vi "总磷总氮MB_api.vi"(6 "Slave ID":u8=1, 7 "STEP":enum16{"open", "read", "write", "close"}(ring)=enum."read", 8 "Error in":errorcluster caption="Error in (no error)", 9 "values":u16[](array[numeric]), 10 "quantity":u16, 11 "starting address":u16 format="%04xH") -> (0 "error out":errorcluster, 2 "MB session out":refnum<class "MB_Master.lvclass">, 3 "Registers":u16[](array[numeric]))   [LabVIEW 2016, in "斯坦道总磷.lvlib"]
uses:
  <vilib>/Plasmionique/MB Master/MB_Master/MB_Master.lvclass
  <vilib>/Plasmionique/MB Master/MB_Master_Serial/MB_Master_Serial.lvclass
  D:/Program Files (x86)/National Instruments/LabVIEW 2016/vi.lib/Plasmionique/MB Master/MB_Master/MB_Master.lvclass
  <vilib>/Plasmionique/MB Master/MB_Master_TCP/MB_Master_TCP.lvclass
  <vilib>/Plasmionique/MB Master/MB Master.lvlib
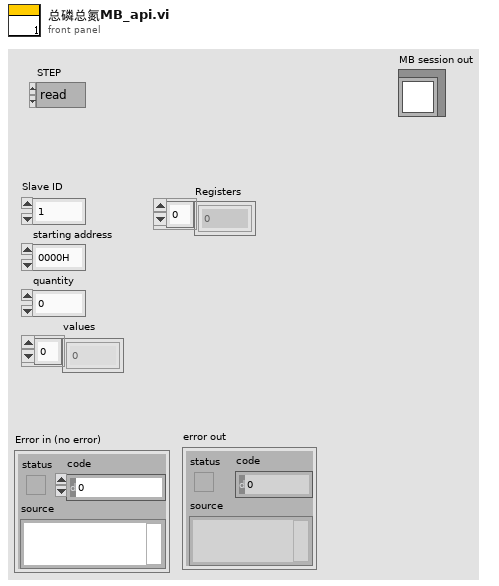
[diagram p1: front panel]
types:
  T1 = cluster{"baud rate (bps)":u32, "stop bits":u16, "parity":u16, "flow control":u16, "timeout":u32, "retries":i32}
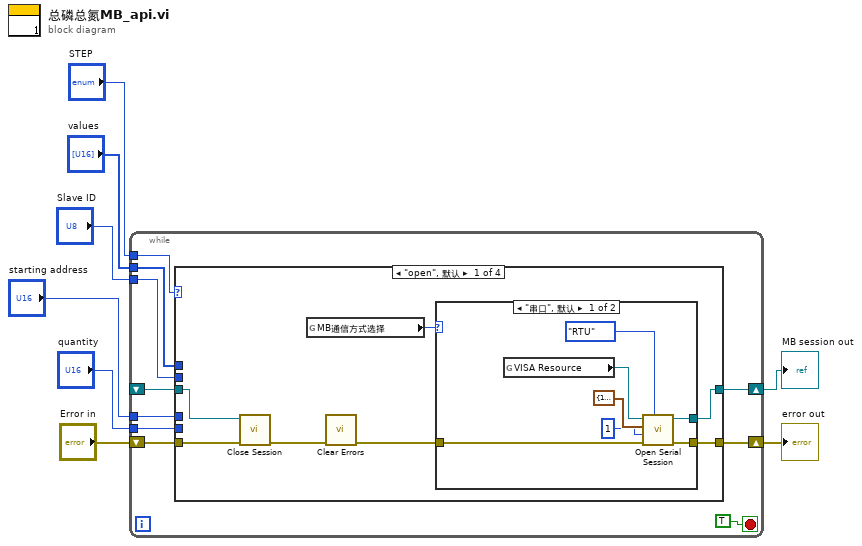
[diagram p0: block diagram]
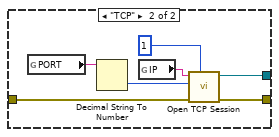
[diagram p2: hidden frame]
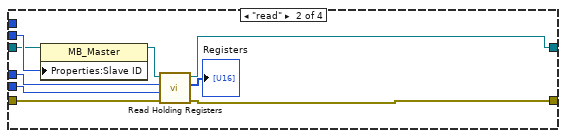
[diagram p3: hidden frame]
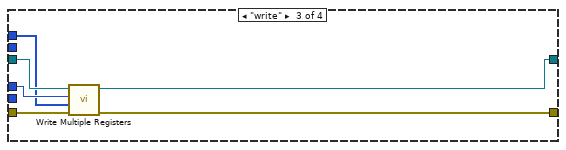
[diagram p4: hidden frame]
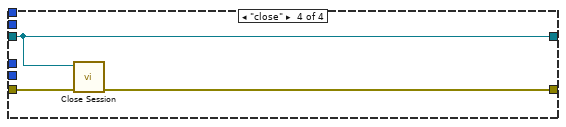
[diagram p5: hidden frame]
diagram:
  n1 = while {
    shift-right: [w9] -> w1
    shift-left: _ -> [w18]
    shift-right: [w10] -> w7
    shift-left: "Error in" -> [w17]
    tunnel: "Slave ID" -> [w16]
    tunnel: "starting address" -> [w15]
    tunnel: "quantity" -> [w14]
    tunnel: "STEP" -> [w13]
    tunnel: "values" -> [w12]
    stop <- TRUE stop-if-true
    n2 = case shown="\"open\", 默认" w13 {
      tunnel: w18 -> [w23 w41 w52 w55]
      tunnel: w17 -> [w22 w48 w54 w57]
      tunnel: [w24 w47 w51 w55] -> w9
      tunnel: [w25 w46 w53 w56] -> w10
      tunnel: w16 -> [_ w44 _ _]
      tunnel: w15 -> [_ w43 w50 _]
      tunnel: w14 -> [_ w42 _ _]
      tunnel: w12 -> [_ _ w49 _]
      frame "open", Default {
        n3 = call-dynamic "Close Session.vi"("error in (no error)"=w22, "MB session in"=w23) -> ("error out"=w21:errorcluster)  [unwired: 9 in]
        n4 = global read "总磷断电保存全局变量.vi" "MB通信方式选择"() -> (w19:enum16{"串口", "TCP"})
        n5 = call <vilib>:"Clear Errors.vi"("error in (no error)"=w21) -> ("error out"=w20:errorcluster)  [unwired: 5 in, 1 out]
        n6 = case shown="\"串口\", 默认" w19 {
          tunnel: [w30 w37] -> w25
          tunnel: [w27 w36] -> w24
          tunnel: w20 -> [w28 w38]
          frame "串口", Default {
            n7 = global read "总磷断电保存全局变量.vi" "VISA Resource"() -> (w26:refnum<visa-resource-name>)
            n8 = call <vilib>:"Open Serial Session.vi"("Mode (RTU)"=enum16{"RTU", "ASCII"}."RTU", "Error in"=w28, "Slave ID"=u8 1, "Serial Config"=T1 {"baud rate (bps)"=115200, "stop bits"=10, "parity"=0, "flow control"=0, "timeout"=1000, "retries"=1}, "VISA Resource"=w26) -> ("Error out"=w30:errorcluster, "MB_Serial session"=w27:refnum<class "MB_Master_Serial.lvclass">)  [unwired: 5 in]
          }
          frame "TCP" {
            n9 = global read "总磷断电保存全局变量.vi" "PORT"() -> (w34:string)
            n10 = Decimal String To Number(string=w34) -> (number=w39:i32)  [unwired: 2 in, 1 out]
            n11 = global read "总磷断电保存全局变量.vi" "IP"() -> (w35:string)
            n12 = call <vilib>:"Open TCP Session.vi"("Slave ID (255)"=u8 1 ("Slave ID"), "error in (no error)"=w38, "Port (502)"=w39, "IP Address"=w35) -> ("error out"=w37:errorcluster, "MB_TCP session"=w36:refnum<class "MB_Master_TCP.lvclass">)  [unwired: 6 in]
          }
        }
      }
      frame "read" {
        n13 = property class="MB_Master"(reference=w41, "Properties:Slave ID"=w44) -> (reference out=w40:refnum<class "MB_Master.lvclass">)  [unwired: 1 in, 1 out]
        n14 = call <vilib>:"Read Holding Registers.vi"("error in (no error)"=w48, "quantity"=w42, "starting address"=w43, "MB session in"=w40) -> ("error out"=w46:errorcluster, "Registers"=→"Registers":u16[], "MB session out"=w47:refnum<class "MB_Master.lvclass">)  [unwired: 5 in]
      }
      frame "write" {
        n15 = call <vilib>:"Write Multiple Registers.vi"("error in (no error)"=w54, "values"=w49, "starting address"=w50, "MB session in"=w52) -> ("error out"=w53:errorcluster, "MB session out"=w51:refnum<class "MB_Master.lvclass">)  [unwired: 6 in]
      }
      frame "close" {
        n16 = call-dynamic "Close Session.vi"("error in (no error)"=w57, "MB session in"=w55) -> ("error out"=w56:errorcluster)  [unwired: 9 in]
      }
    }
  }
  "error out" <- w7
  "MB session out" <- w1
